vi "VCS Set Motor Type.vi"(8 "error in (no error)":errorcluster, 10 "motor type":u16(ring)=10 items=["DC motor"=1, "EC motor (sinus commutated)"=10, "EC motor (block commutated)"=11], 11 "axis in":cluster{"keyHandle":u32, "nodeId":u16}={"keyHandle"=0, "nodeId"=1}) -> (0 "error out":errorcluster, 3 "axis out":cluster{"keyHandle":u32, "nodeId":u16}={"keyHandle"=0, "nodeId"=1})   [LabVIEW 2018]
doc: "With function <B>VCS_SetMotorType</B> the motor type is written."
uses:
  Resources/EposCmd64.dll
  Resources/EposCmd.dll
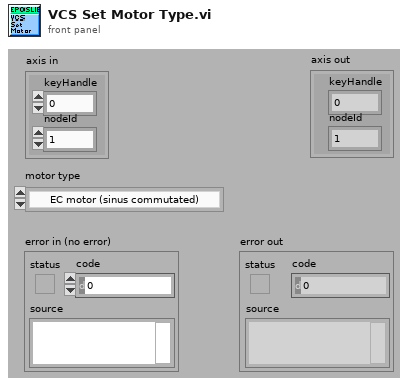
[diagram p1: front panel]
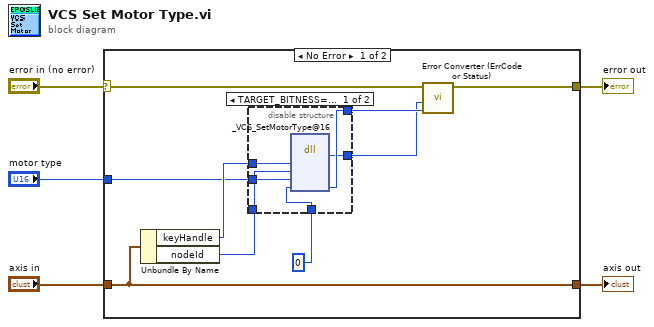
[diagram p0: block diagram]
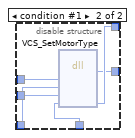
[diagram p2: hidden frame]
diagram:
  n1 = case shown="No Error" "error in (no error)" {
    selector: "error in (no error)" -> [w12 w27]
    tunnel: "axis in" -> [w14 w28]
    tunnel: [w14 w28] -> w4
    tunnel: [w13 w27] -> w3
    tunnel: "motor type" -> [w6 _]
    frame No Error {
      n2 = Unbundle By Name(w14) -> ("keyHandle"=w10:u32, "nodeId"=w9:u16)
      n3 = disable-structure shown="TARGET_BITNESS==32, Standard" {
        disable-tunnel: u32 0 ("pErrorCode") -> [w20 w26]
        disable-tunnel: w10 -> [w19 w25]
        disable-tunnel: w9 -> [w18 w24]
        disable-tunnel: [w17 w23] -> w8
        disable-tunnel: [w16 w22] -> w7
        disable-tunnel: w6 -> [w15 w21]
        frame condition #0 (active) {
          n4 = dll-call lib="C:/Projeto em LabVIEW/EPOS-LabVIEW-Instrument-Driver-En/LabVIEW/maxon EPOS/Resources/EposCmd.dll" fn="_VCS_SetMotorType@16"("KeyHandle"=w19, "NodeId"=w18, "MotorType"=w15, "pErrorCode"=w20) -> ("Rückgabetyp"=w16:i32, "pErrorCode"=w17:u32)  [unwired: 6 in, 2 out]
        }
        frame condition #1 {
          n5 = dll-call lib="C:/Temp/Tests/LabVIEW/maxon EPOS/Resources/EposCmd64.*" fn="VCS_SetMotorType" ("EposCmd.dll:_VCS_SetMotorType@16")("KeyHandle"=w25, "NodeId"=w24, "MotorType"=w21, "pErrorCode"=w26) -> ("Rückgabetyp"=w22:i32, "pErrorCode"=w23:u32)  [unwired: 6 in, 2 out]
        }
      }
      n6 = call "Error Converter (ErrCode or Status).vi"("error code"=w8, "return type"=w7, "error in (no error)"=w12) -> ("error out"=w13:errorcluster)  [unwired: 7 in]
    }
    frame Error {
    }
  }
  "error out" <- w3
  "axis out" <- w4
